vi "Return Notifier.vi"(8 "error in":errorcluster, 9 "Input Data":variant, 10 "Return Data":variant) -> (0 "error out":errorcluster, 1 "found":bool)   [LabVIEW 2013, in "命令队列.lvlib"]
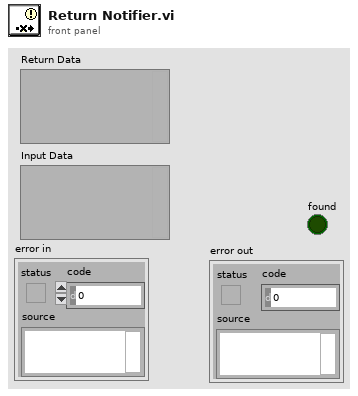
[diagram p1: front panel]
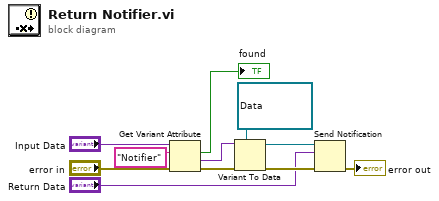
[diagram p0: block diagram]
diagram:
  n1 = Get Variant Attribute(Variant="Input Data", name="Notifier", error in="error in") -> (found=→"found":bool, value=w4:variant, error out=w9:errorcluster)  [unwired: 1 in, 1 out]
  n2 = Variant To Data(error in=w9, type=refnum<notifier> refnum ("notifier out"), Variant=w4) -> (data=w5:refnum<notifier>, error out=w10:errorcluster)
  n3 = Send Notification(notification="Return Data", notifier=w5, error in (no error)=w10) -> (error out=→"error out":errorcluster)  [unwired: 1 out]
